vi "PH_GUI_Class.Delete GUI.vi"(0 "VI in":refnum<vi>, 5 "error in (no error)":errorcluster) -> (14 "VI out":refnum<vi>, 19 "error out":errorcluster)   [LabVIEW 2014, in "PH_GUI_Class.lvlib"]
uses:
  PH_GUI_Class.lvlib
  CS_Core/CSObj/CSObj.lvlib
  PH_Common/PH_Common.lvlib
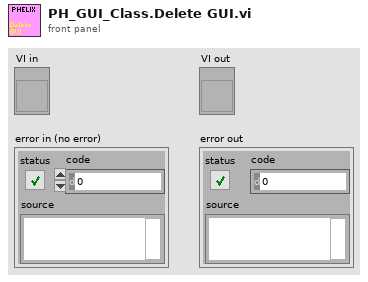
[diagram p1: front panel]
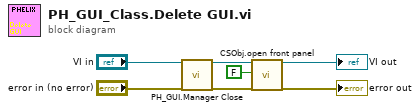
[diagram p0: block diagram]
diagram:
  n1 = call "PH_GUI.Manager Close.vi"("i ref in"="VI in", "error in"="error in (no error)") -> ("i ref out"=w7:refnum<vi>, "error out"=w5:errorcluster)  [unwired: 16 in]
  n2 = call "CSObj.open front panel.vi"("i ref in"=w7, "frontPanelOpen"=FALSE ("front panel open"), "error in (no error)"=w5) -> ("i ref out"=→"VI out":refnum<vi>, "error out"=→"error out":errorcluster)  [unwired: 15 in]
